vi "Button_Create.vi"(0 "reference in":refnum<class "Button.lvclass">, 1 "Text":string, 2 "Override size":cluster{"Width":i16, "Height":i16}, 5 "error in (no error)":errorcluster) -> (14 "reference out":refnum<class "Button.lvclass">, 19 "error out":errorcluster)   [LabVIEW 2019, in "Button.lvclass"]
uses:
  Button.lvclass
  C:/Users/Taylor.Hillegeist/OneDrive - Ultra/LabVIEW/Pgui2/Pgui_Obj_class/Pgui_Obj.lvclass
  Pgui_Obj_class/Pgui_Obj.lvclass
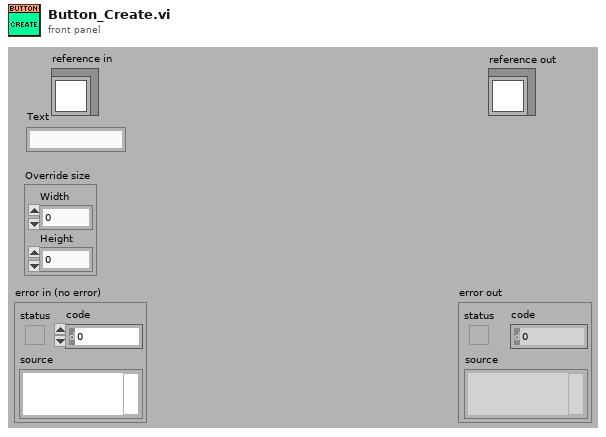
[diagram p1: front panel]
types:
  T1 = typedef "Pgui_Button.lvclass/ObjectAttributes.ctl" = cluster{"Text":string, "Override size":cluster{"Width":i16, "Height":i16}}
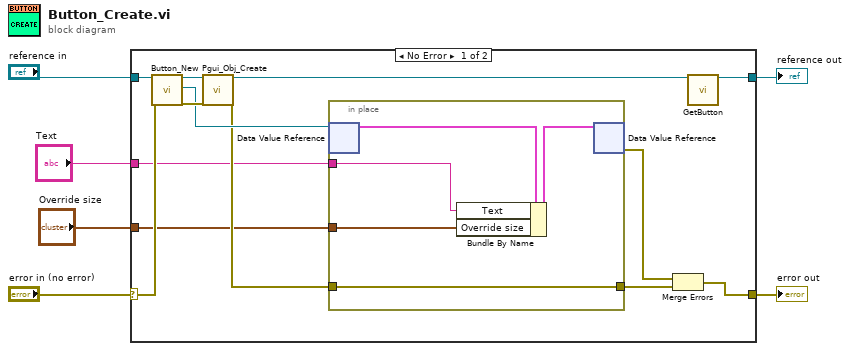
[diagram p0: block diagram]
diagram:
  n1 = case shown="No Error" "error in (no error)" {
    selector: "error in (no error)" -> [w18 w26]
    tunnel: [w16 w26] -> w5
    tunnel: "reference in" -> [w19 w25]
    tunnel: [w7 w25] -> w3
    tunnel: "Text" -> [w10 _]
    tunnel: "Override size" -> [w9 _]
    frame No Error {
      n2 = call "Button_New.vi"("reference in"=w19, "error in (no error)"=w18) -> ("reference out"=w15:refnum<class "Button.lvclass">, "DVRRefOut"=w13:refnum<data-value>, "error out"=w14:errorcluster)  [unwired: 14 in, 1 out]
      n3 = call "Pgui_Obj_Create.vi"("reference in"=w15, "error in (no error)"=w14) -> ("reference out"=w8:refnum<class "Button.lvclass">, "error out"=w12:errorcluster)  [unwired: 16 in]
      n4 = in-place {
        in-place-border: w12 -> [w22]
        in-place-border: [w22] -> w11
        in-place-border: w10 -> [w21]
        in-place-border: w9 -> [w20]
        n5 = in-place-dvr #1(w13) -> (w23:T1)  [unwired: 1 out]
        n6 = Bundle By Name(cluster=w23, "Text"=w21, "Override size"=w20) -> (w24:T1)
        n7 = in-place-dvr #1(w24) -> (w17:errorcluster)  [unwired: 1 out]
      }
      n8 = Merge Errors(w17, w11) -> (w16:errorcluster)
      n9 = call-dynamic "GetButton.vi"("reference in"=w8) -> ("reference out"=w7:refnum<class "Button.lvclass">)  [unwired: 17 in, 1 out]
    }
    frame Error {
    }
  }
  "error out" <- w5
  "reference out" <- w3
